vi "BPF.vi"(1 "enable":bool, 2 "in":dbl[](array[numeric]), 4 "fc":dbl) -> (6 "out":dbl[](array[numeric]))   [LabVIEW 2015]
uses:
  <vilib>/Analysis/3filter.llb/Filter Passband Type.ctl
  <vilib>/Analysis/3filter.llb/Butterworth Filter (DBL).vi
  <vilib>/Analysis/NI_AALBase.lvlib
panel:
  in  "f_max":dbl
  in  "sampling freq: fs":dbl=1.0 format="%0.2f"
  # "Bandpass filter"
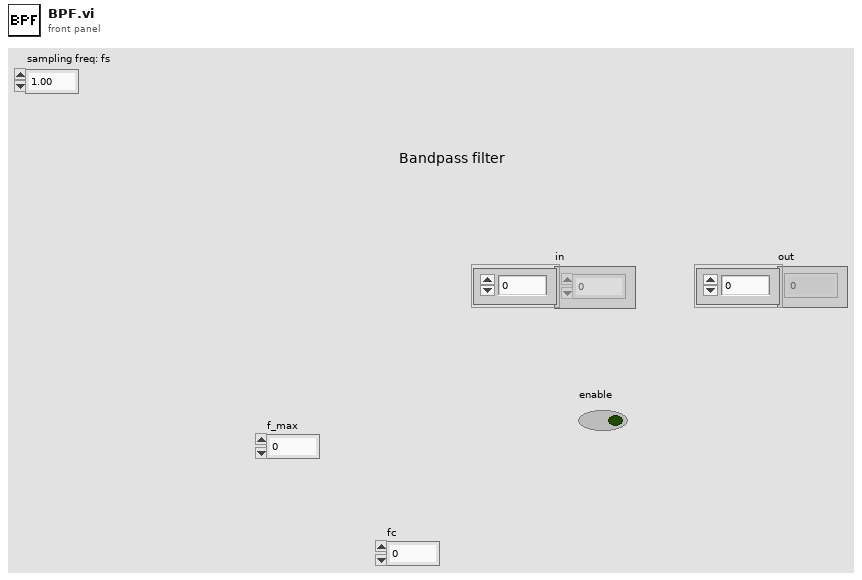
[diagram p1: front panel]
types:
  T1 = typedef "NI_AALBase.lvlib/Filter Passband Type.ctl" = enum32{"Lowpass", "Highpass", "Bandpass", "Bandstop"}
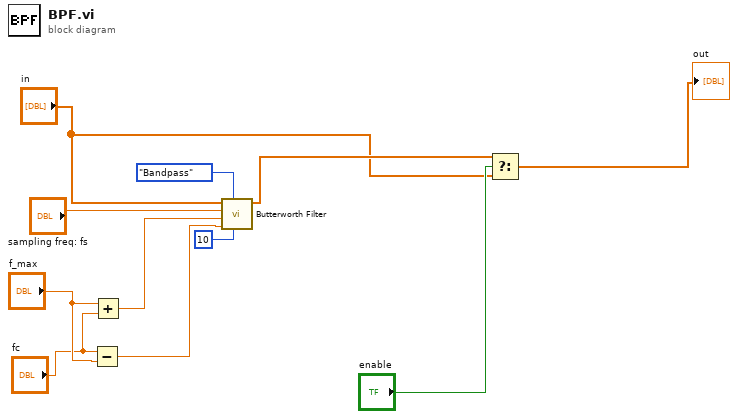
[diagram p0: block diagram]
diagram:
  n1 = Subtract(x="fc", y="f_max") -> (x-y=w5:dbl)
  n2 = Add(x="f_max", y="fc") -> (x+y=w6:dbl)
  n3 = call-poly <vilib>:"Butterworth Filter.vi"("order"=10, "filter type"=Filter_Passband_Type."Bandpass", "low cutoff freq: fl"=w5, "high cutoff freq: fh"=w6, "sampling freq: fs"="sampling freq: fs", "X"="in") -> ("Filtered X"=w3:dbl[])  [unwired: 2 in, 1 out]
  n4 = Select(t=w3, s="enable", f="in") -> (s? t:f=→"out":dbl[])
